vi "String Example.vi"() -> ()   [LabVIEW 2011]
panel:
  out "result string 2":string
  out "result string":string
  out "concatenated string":string
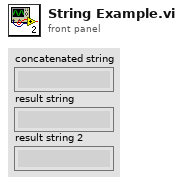
[diagram p1: front panel]
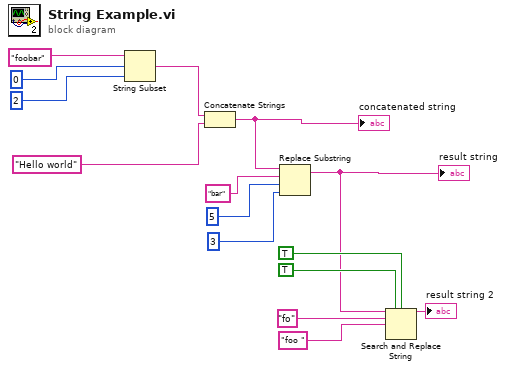
[diagram p0: block diagram]
diagram:
  n1 = String Subset(string="foobar", offset (0)=0, length (rest)=2 ("length (rest)")) -> (substring=w11:string)
  n2 = Concatenate Strings(w11, "Hello world") -> (w10:string)
  "concatenated string" <- w10
  n3 = Replace Substring(2:3 ("length (len. of substring)"), 3:5 ("offset (0)"), 4:"bar", 5:w10) -> (1:w4:string)  [unwired: 1 out]
  "result string" <- w4
  n4 = Search and Replace String(replace all?=TRUE ("replace all? (F)"), case sensitive?=TRUE ("ignore case? (F)"), input string=w4, search string="fo", replace string="foo " ("replace string (\"\")")) -> (result string=→"result string 2":string)  [unwired: 3 in, 3 out]
